vi "IF2_DeviceConfiguration.vi"(8 "error in":errorcluster, 11 "TCP  in":refnum<k5>) -> (0 "error out":errorcluster, 3 "TCP Network Connection out":refnum<k5>)   [LabVIEW 2015, in "IF2_Reader.lvlib"]
uses:
  IF2_Reader.lvlib
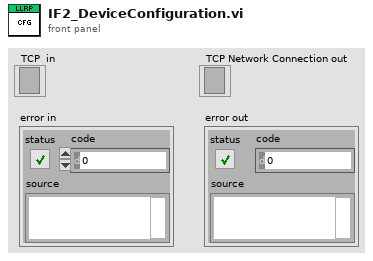
[diagram p1: front panel]
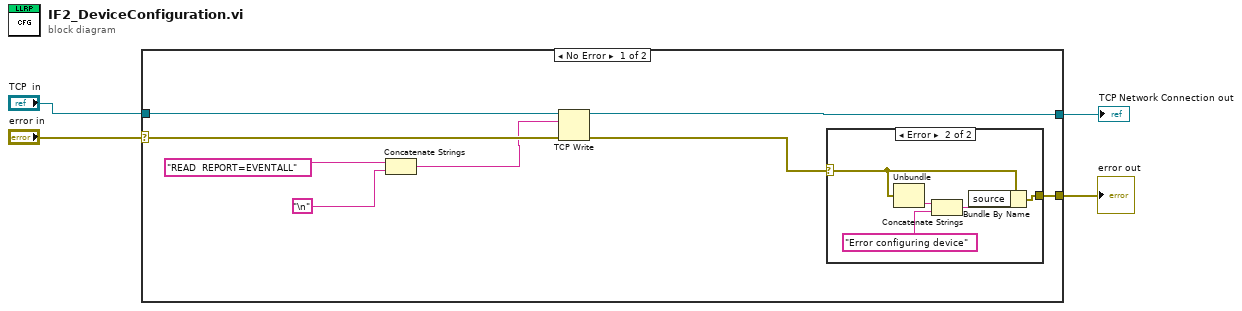
[diagram p0: block diagram]
diagram:
  n1 = case shown="No Error" "error in" {
    selector: "error in" -> [w8 w19]
    tunnel: "TCP  in" -> [w9 w20]
    tunnel: [w11 w20] -> w4
    tunnel: [w12 w19] -> w1
    frame No Error {
      n2 = Concatenate Strings("READ  REPORT=EVENTALL" ("data in"), "\n") -> (w5:string)
      n3 = TCP Write(connection ID=w9, data in=w5, error in (no error)=w8) -> (connection ID out=w11:refnum<k5>, error out=w10:errorcluster)  [unwired: 2 out]
      n4 = case shown="Error" w10 {
        selector: w10 -> [w13 w18]
        tunnel: [w13 w17] -> w12
        frame No Error {
        }
        frame Error {
          n5 = Unbundle(w18) -> ("source"=w16:string)  [unwired: 2 out]
          n6 = Concatenate Strings(w16, "Error configuring device" ("string")) -> (w15:string)
          n7 = Bundle By Name(cluster=w18, "source"=w15) -> (w17:errorcluster)
        }
      }
    }
    frame Error {
    }
  }
  "TCP Network Connection out" <- w4
  "error out" <- w1
